vi "MeasurementServer_SetResponse_Query.vi"(0 "gRPCid":T1, 1 "message":string, 2 "status":i32, 3 "error in (no error)":errorcluster) -> (10 "error out":errorcluster)   [LabVIEW 2019, in "labview-grpc-measurement-server.lvlib"]
uses:
  labview-grpc-measurement-server.lvlib
  MeasurementServer_gRPCid.ctl
  MeasurementServer_QueryResponse.ctl
  home/lvuser/liblabview_measurement_server.so
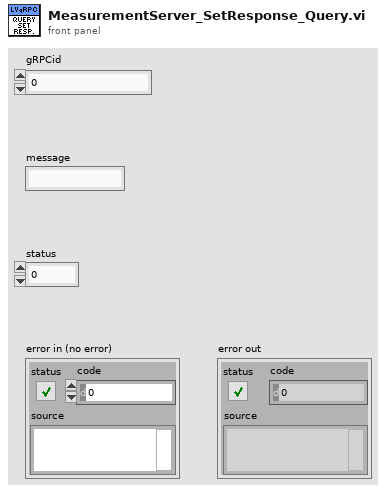
[diagram p1: front panel]
types:
  T1 = typedef "labview-grpc-measurement-server.lvlib/MeasurementServer_gRPCid.ctl" = u64
  T2 = typedef "labview-grpc-measurement-server.lvlib/MeasurementServer_QueryResponse.ctl" = cluster{"message":string, "status":i32}
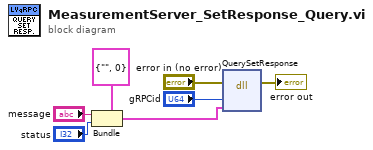
[diagram p0: block diagram]
diagram:
  n1 = Bundle(cluster=T2 {"message"="", "status"=0} ("QueryResponse"), "message"="message", "status"="status") -> (w3:T2)
  n2 = dll-call lib="home/lvuser/liblabview_measurement_server.so" fn="QuerySetResponse"(error in="error in (no error)", "id"="gRPCid", "data"=w3) -> (error out=→"error out":errorcluster)  [unwired: 5 in, 1 out]
